vi "LocateConfigFile.vi"(8 "error in (no error)":errorcluster, 11 "SMO.UI.MAUI in":refnum<class "MAUI.lvclass">) -> (0 "error out":errorcluster, 2 "Config File Path":path, 3 "SMO.UI.MAUI out":refnum<class "MAUI.lvclass">)   [LabVIEW 2019, in "MAUI.lvclass"]
doc: "Locates the configuration file path. If MAUI is used in an inheritance relationship, this will be based on the childs name. If MAUI is used in composition relationship, it will be based on either a path provided, or as an application name."
uses:
  MAUI.lvclass
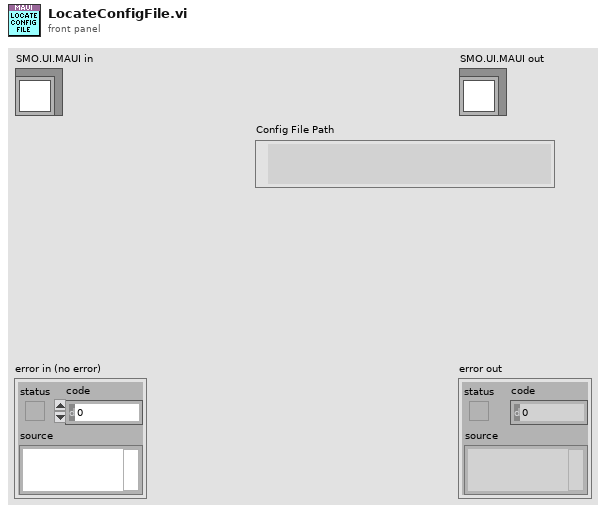
[diagram p1: front panel]
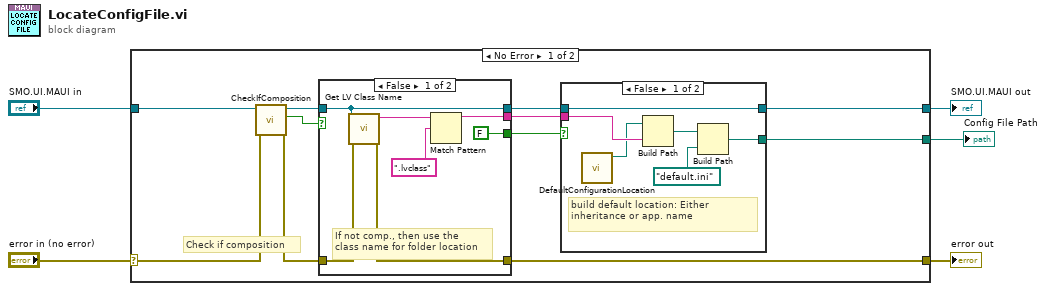
[diagram p0: block diagram]
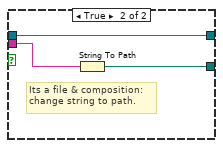
[diagram p2: hidden frame]
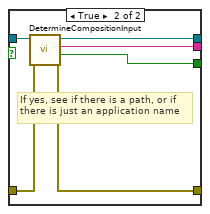
[diagram p3: hidden frame]
diagram:
  n1 = case shown="No Error" "error in (no error)" {
    selector: "error in (no error)" -> [w16 w40]
    tunnel: [w6 w40] -> w4
    tunnel: [w11 w39] -> w2
    tunnel: "SMO.UI.MAUI in" -> [w7 w39]
    tunnel: [w8 _] -> w1
    frame No Error {
      # "Check if composition"
      n2 = call "CheckIfComposition.vi"("error in (no error)"=w16, "SMO.UI.MAUI in"=w7) -> ("error out"=w13:errorcluster, "Is Composition?"=w14:bool, "SMO.UI.MAUI out"=w15:refnum<class "MAUI.lvclass">)  [unwired: 7 in]
      n3 = case shown="False" w14 {
        tunnel: w15 -> [w32 w38]
        tunnel: [w32 w37] -> w12
        tunnel: w13 -> [w27 w33]
        tunnel: [w28 w34] -> w6
        tunnel: [w29 w36] -> w9
        tunnel: [FALSE w35] -> w10
        frame False {
          # "If not comp., then use the \nclass name for folder location"
          n4 = call <vilib>:"Get LV Class Name.vi"("error in (no error)"=w27, "object"=w32) -> ("error out"=w28:errorcluster, "class name"=w30:string)  [unwired: 8 in]
          n5 = Match Pattern(string=w30, regular expression=".lvclass") -> (before substring=w29:string)  [unwired: 1 in, 3 out]
        }
        frame True {
          # "If yes, see if there is a path, or if\nthere is just an application name"
          n6 = call "DetermineCompositionInput.vi"("error in (no error)"=w33, "SMO.UI.MAUI in"=w38) -> ("error out"=w34:errorcluster, "Is Path?"=w35:bool, "Composition Input"=w36:string, "SMO.UI.MAUI out"=w37:refnum<class "MAUI.lvclass">)  [unwired: 5 in, 1 out]
        }
      }
      n7 = case shown="False" w10 {
        tunnel: w12 -> [w22 w25]
        tunnel: [w22 w25] -> w11
        tunnel: w9 -> [w21 w23]
        tunnel: [w17 w24] -> w8
        frame False {
          # "build default location: Either inheritance or app. name"
          n8 = call "DefaultConfigurationLocation.vi"() -> ("DefaultConfigLocation"=w20:path)  [unwired: 11 in]
          n9 = Build Path(base path=w20, name or relative path=w21) -> (appended path=w19:path)
          n10 = Build Path(base path=w19, name or relative path=path "default.ini") -> (appended path=w17:path)
        }
        frame True {
          # "Its a file & composition:\nchange string to path."
          n11 = String To Path(string=w23) -> (path=w24:path)
        }
      }
    }
    frame Error {
    }
  }
  "error out" <- w4
  "SMO.UI.MAUI out" <- w2
  "Config File Path" <- w1
